vi "FRCts20_Backend_SetSingleTeam.vi"(6 "Message Attributes":T4, 8 "error in (no error)":errorcluster, 10 "Team Dfn":string, 11 "Engine_Refnums":T1) -> (0 "error out":errorcluster)   [LabVIEW 2014, in "FRCts20_Backend_Engine_Deprecated.lvlib"]
doc: "Despite the name, this VI actually just adds a team with the provided team data or updates (really replaces) a team with a given team number with new data for that team with the same team number."
uses:
  FRCts20_Backend_Engine_Deprecated.lvlib
  FRCts20_Backend_FGVOperation.ctl
  FRCts20_Backend_Engine.lvlib
  Dependencies/Keyed Array/KeyedArray.ctl
  Dependencies/Keyed Array/Tools_KeyedArray.lvlib
  Dependencies/AMC/_SubVIs/TypeDefs/Message.ctl
  Dependencies/AMC/AMC.lvlib
  Dependencies/AMC/_SubVIs/TypeDefs/Message Queue.ctl
  FRCts20_Backend_EngineRefnums.ctl
  <vilib>/addons/database/Connection.llb/Conn ObjectReference.ctl
  <vilib>/addons/database/NI_Database_API.lvlib
  INI_Accessor/FRCts20_Backend_INI Controller.lvclass
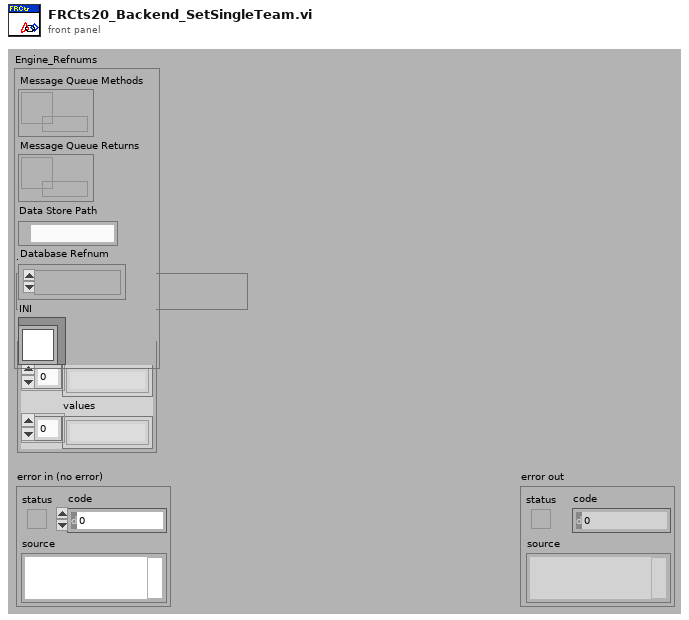
[diagram p1: front panel]
types:
  T1 = typedef "FRCts20_Backend_Engine.lvlib/FRCts20_Backend_EngineRefnums.ctl" = cluster{"Message Queue Methods":T2, "Message Queue Returns":T2, "Data Store Path":path, "Database Refnum":T3, "INI":refnum<class "FRCts20_Backend_INI Controller.lvclass">}
  T2 = typedef "AMC.lvlib/Message Queue.ctl" = refnum<queue>
  T3 = typedef "NI_Database_API.lvlib/Conn ObjectReference.ctl" = refnum<k1>
  T4 = typedef "Tools_KeyedArray.lvlib/KeyedArray.ctl" = cluster{"keys":string[], "values":string[]}
  T5 = typedef "FRCts20_Backend_Engine.lvlib/FRCts20_Backend_FGVOperation.ctl" = enum16{"Initialize", "EnqueueMessage", "EnqueueDataReturn", "FlushMessage", "FlushDataReturn"}
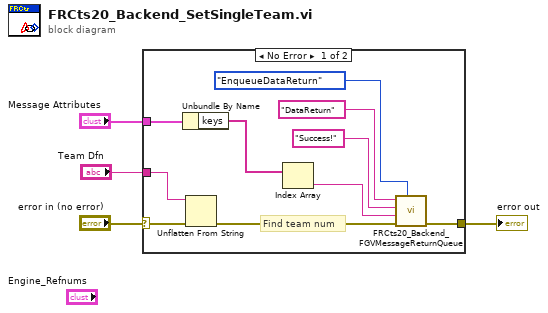
[diagram p0: block diagram]
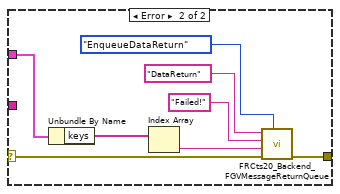
[diagram p2: hidden frame]
diagram:
  n1 = case shown="No Error" "error in (no error)" {
    selector: "error in (no error)" -> [w7 w16]
    tunnel: [w14 w15] -> w3
    tunnel: "Team Dfn" -> [w6 _]
    tunnel: "Message Attributes" -> [w10 w18]
    frame No Error {
      # "Find team num"
      n2 = Unbundle By Name(w10) -> ("keys"=w9:string[])
      n3 = Unflatten From String(binary string=w6, error in (no error)=w7) -> (error out=w5:errorcluster)  [unwired: 3 in, 2 out]
      n4 = Index Array(array=w9) -> (element=w8:string)  [unwired: 1 in]
      n5 = call "FRCts20_Backend_FGVMessageReturnQueue.vi"("Operation"=FRCts20_Backend_FGVOperation."EnqueueDataReturn", "error in (no error)"=w5, "Key"=w8, "Message Value"="Success!" ("Message Name"), "Message Name"="DataReturn") -> ("error out"=w14:errorcluster)  [unwired: 3 in, 1 out]
    }
    frame Error {
      n6 = Unbundle By Name(w18) -> ("keys"=w19:string[])
      n7 = Index Array(array=w19) -> (element=w17:string)  [unwired: 1 in]
      n8 = call "FRCts20_Backend_FGVMessageReturnQueue.vi"("Operation"=FRCts20_Backend_FGVOperation."EnqueueDataReturn", "error in (no error)"=w16, "Key"=w17, "Message Value"="Failed!" ("Message Name"), "Message Name"="DataReturn") -> ("error out"=w15:errorcluster)  [unwired: 3 in, 1 out]
    }
  }
  "error out" <- w3
